vi "Remove Trailing Zeros.vi"(1 "Floating Point Number":string) -> (0 "Remove Trailing Zeros":string)   [LabVIEW 2020, in "eec EST 300.lvlib"]
doc: "This utility vi removes trailing zeros from the ASCII representation of a floating point number."
uses:
  <instrlib>/eec EST 300/eec EST 300.lvlib
panel:
  # "This assumes that the floating point number is at the\nend of the string."
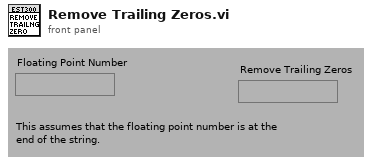
[diagram p1: front panel]
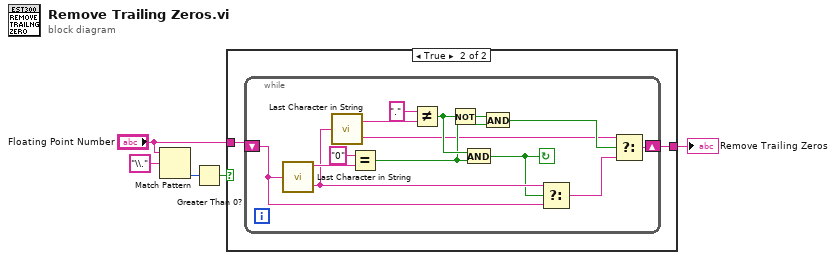
[diagram p0: block diagram]
diagram:
  n1 = Match Pattern(string="Floating Point Number", regular expression="\\.") -> (offset past match=w3:i32)  [unwired: 1 in, 3 out]
  n2 = Greater Than 0?(x=w3) -> (x > 0?=w1:bool)
  n3 = case shown="True" w1 {
    tunnel: [w6 w8] -> w5
    tunnel: "Floating Point Number" -> [w6 w7]
    frame False {
    }
    frame True {
      n4 = while {
        shift-left: w7 -> [w17]
        shift-right: [w9] -> w8
        stop <- w16 continue-if-true
        n5 = call <instrlib>:"Last Character in String.vi"("Input  String (empty)"=w17) -> ("Last Character"=w22:string, "Rest of String"=w18:string)
        n6 = call <instrlib>:"Last Character in String.vi"("Input  String (empty)"=w18) -> ("Last Character"=w20:string, "Rest of String"=w10:string)
        n7 = Equal?(x="0", y=w22) -> (x = y?=w14:bool)
        n8 = Not Equal?(x="." ("y"), y=w20) -> (x != y?=w15:bool)
        n9 = Not(x=w15) -> (.not. x?=w13:bool)
        n10 = And(x=w15, y=w14) -> (x .and. y?=w16:bool)
        n11 = And(x=w13, y=w14) -> (x .and. y?=w12:bool)
        n12 = Select(t=w18, s=w16, f=w17) -> (s? t:f=w11:string)
        n13 = Select(t=w10, s=w12, f=w11) -> (s? t:f=w9:string)
      }
    }
  }
  "Remove Trailing Zeros" <- w5
